vi "Increment_Variables_noise.vi"(8 "error in 2":errorcluster, 10 "Dummy Variable":dbl=1.0, 11 "Sound":waveform(dbl)[](array[waveform])) -> (0 "error IO":errorcluster, 2 "Dummy Variable Array":dbl[](array[numeric]), 3 "Time Stamp":timestamp[](array[timestamp]))   [LabVIEW 2016]
uses:
  <vilib>/Utility/error.llb/DialogType.ctl
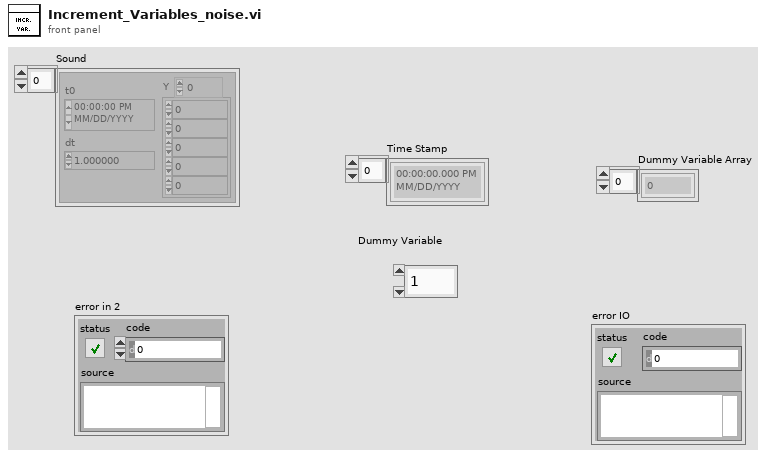
[diagram p1: front panel]
types:
  T1 = typedef "DialogType.ctl" = u16
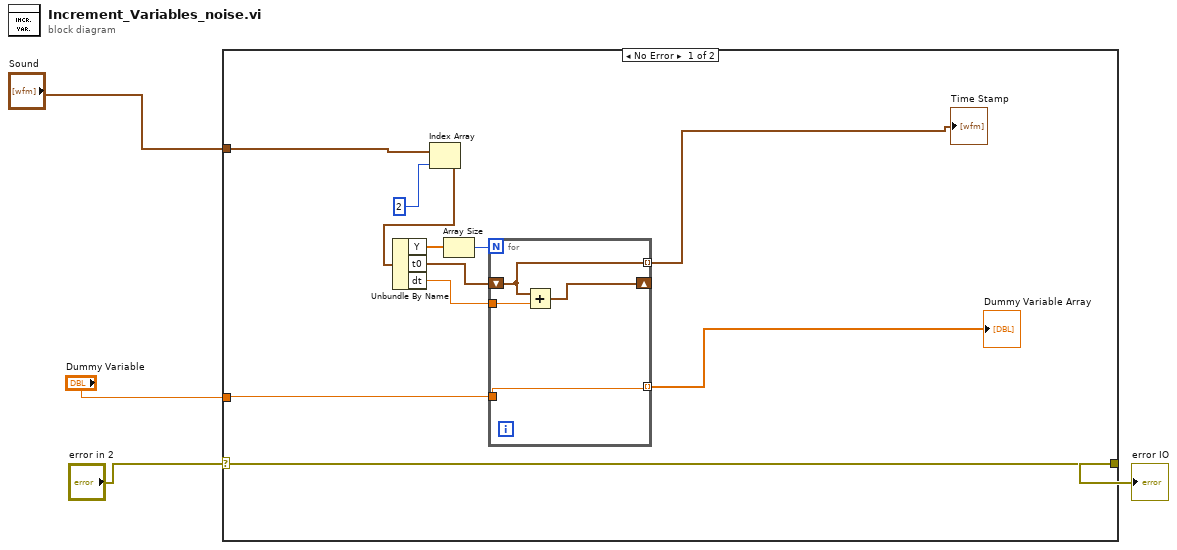
[diagram p0: block diagram]
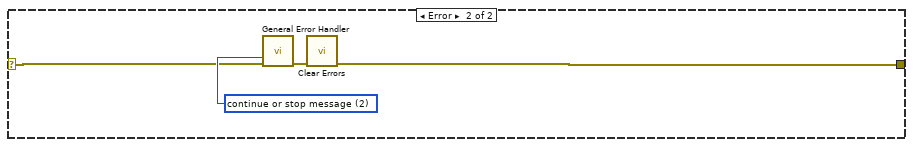
[diagram p2: hidden frame]
diagram:
  n1 = case shown="No Error" "error in 2" {
    selector: "error in 2" -> [w8 w21]
    tunnel: "Dummy Variable" -> [w15 _]
    tunnel: "Sound" -> [w5 _]
    tunnel: [w8 w20] -> w2
    frame No Error {
      n2 = Index Array(array=w5, index=2) -> (element=w13:waveform(dbl))
      n3 = Unbundle By Name(w13) -> ("Y"=w9:dbl[], "t0"=w11:timestamp, "dt"=w12:dbl)
      n4 = Array Size(array=w9) -> (size(s)=w10:i32)
      n5 = for {
        N: w10 -> [_]
        tunnel: w12 -> [w19]
        shift-right: [w18] -> _
        shift-left: w11 -> [w17]
        tunnel: [w17] -> w6 mode=indexing
        tunnel: [w16] -> w7 mode=indexing
        tunnel: w15 -> [w16]
        n6 = Add(x=w17, y=w19) -> (x+y=w18:timestamp)
      }
      "Time Stamp" <- w6
      "Dummy Variable Array" <- w7
    }
    frame Error {
      w22 = T1 2 items=["no dialog", "OK message", "continue or stop message", "OK message + warnings", "continue/stop + warnings"] ("type of dialog (OK msg:1)")
      n7 = call <vilib>:"General Error Handler.vi"("type of dialog (OK msg:1)"=w22, "error in (no error)"=w21) -> ("error out"=w23:errorcluster)  [unwired: 9 in, 4 out]
      n8 = call <vilib>:"Clear Errors.vi"("error in (no error)"=w23) -> ("error out"=w20:errorcluster)  [unwired: 5 in, 1 out]
    }
  }
  "error IO" <- w2
